vi "Scale Input Pressure.vi"(9 "Pressure (V)":dbl) -> (1 "Pressure (psi atm)":dbl)   [LabVIEW 2013]
doc: "This sub-VI scales the pressure read by our pressure sensor (volts) to atmospheric psi"
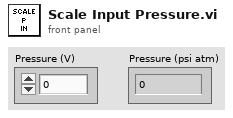
[diagram p1: front panel]
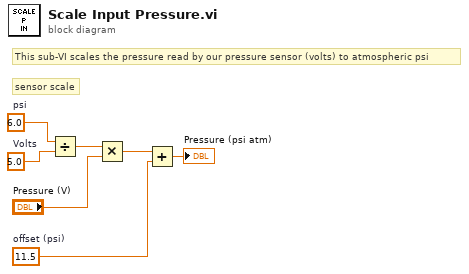
[diagram p0: block diagram]
diagram:
  w6 = 11.5  # offset (psi)
  w2 = 5.0  # Volts
  w1 = 6.0  # psi
  # "sensor scale"
  # "This sub-VI scales the pressure read by our pressure sensor (volts) to atmospheric psi"
  n1 = Divide(x=w1, y=w2) -> (x/y=w3:dbl)
  n2 = Multiply(x=w3, y="Pressure (V)") -> (x*y=w5:dbl)
  n3 = Add(x=w5, y=w6) -> (x+y=→"Pressure (psi atm)":dbl)
